vi "SENS_SEGM_POW_LEV.vi"(0 "VISA IN":refnum<visa-resource-name>, 1 "Segment":i32, 2 "Port":i32, 3 "Power Level":i32, 5 "error in":errorcluster, 7 "Channel":i32) -> (14 "VISA Out":refnum<visa-resource-name>, 19 "error out":errorcluster)   [LabVIEW 2018, in "PNA-X.lvlib"]
doc: "SENSe<cnum>:SEGMent<snum>:POWer[<port>][:LEVel] <num> \n1810\n\n(Read-Write) Sets the Port Power level for the specified sweep segment. First set \nSENS:SEGM:POW:CONTrol ON. \nWhen port power is Coupled, setting port power for one port will apply port power for all source \nports. \nAll subsequent segments that are added assume the new Power Level value. \nParameters \n<cnum> Any existing channel number. If unspecified, value is set to 1 \n<snum> Segment number to modify. Choose any existing segment number. \n<port> Port number of the source. If unspecified, value is set to 1. \n<num> Power level. \nNote: The range of settable power values depends on the PNA model and if \nsource attenuators are installed. To determine the range of values, send \nSOUR:POW? MAX and SOUR:POW? MIN. (SOUR:POW:ATT:AUTO must \nbe set to ON). \nActual achievable leveled power depends on frequency. \nExamples SENS:SEGM:POW 0 \nsense2:segment2:power1:level -10 \nQuery Syntax SENSe<cnum>:SEGMent<snum>:POWer[<port>][:LEVel]? \nReturn Type Numeric \nDefault 0"
uses:
  PNA-X.lvlib
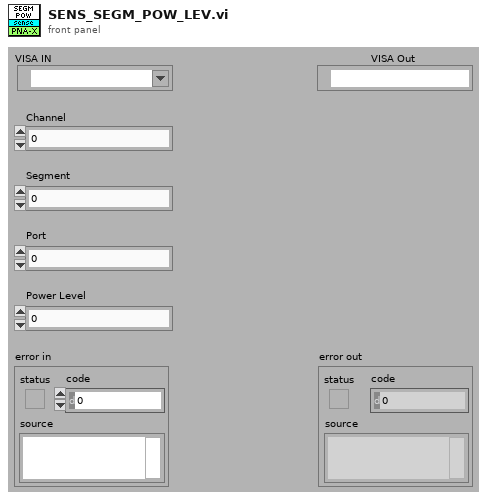
[diagram p1: front panel]
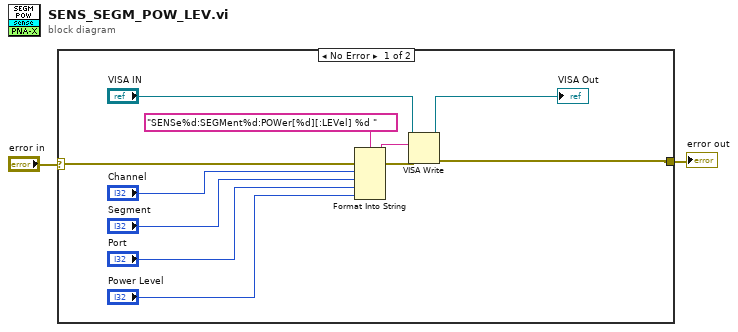
[diagram p0: block diagram]
diagram:
  n1 = case shown="No Error" "error in" {
    selector: "error in" -> [w13 w14]
    tunnel: [w8 w14] -> w1
    frame No Error {
      n2 = Format Into String(format string="SENSe%d:SEGMent%d:POWer[%d][:LEVel] %d " ("Cmdline"), error in=w13, "Channel", "Segment", "Port", "Power Level") -> (resulting string=w11:string, error out=w12:errorcluster)  [unwired: 1 in]
      n3 = VISA Write(VISA resource name="VISA IN", write buffer=w11, error in (no error)=w12) -> (VISA resource name out=→"VISA Out":refnum<visa-resource-name>, error out=w8:errorcluster)  [unwired: 1 out]
    }
    frame Error {
    }
  }
  "error out" <- w1
